vi "Begin.vi"() -> (0 "error out":errorcluster)   [LabVIEW 2013]
doc: "Called before other user functions, this VI is expected to open initial I/O refnums, load in file data, and do all program initialization. Notice that the <B>error out</B> terminal is simply used for data flow. Wiring it to other structures or subVIs ensures that this VI runs first."
uses:
  <vilib>/Rock Robotics/WPI/DriverStation/WPI_DriverStationRobotMode2.ctl
  <vilib>/Rock Robotics/WPI/Relay/WPI_RelayDirection.ctl
  <vilib>/Rock Robotics/SystemInterfaces/Typedef/FPGA_TypedefDigitalModule.ctl
  <vilib>/Rock Robotics/WPI/SafetyOutput/WPI_SafetyOutputConfigMenu.ctl
  <vilib>/Rock Robotics/WPI/Joystick/WPI_JoystickDeviceEnum.ctl
  <vilib>/Rock Robotics/SystemInterfaces/DIO/FPGA_DIOChannel.ctl
  <vilib>/Rock Robotics/WPI/Encoder/WPI_EncoderType.ctl
  <vilib>/Rock Robotics/SystemInterfaces/AI/FPGA_AIGyroChannel.ctl
  <vilib>/Rock Robotics/SystemInterfaces/Typedef/FPGA_TypedefAnalogModuleForGyro.ctl
  <vilib>/Rock Robotics/SystemInterfaces/DIO/FPGA_DIORelayChannel.ctl
  <vilib>/Rock Robotics/WPI/CAN/Jaguar/SubVIs/WPI_CANJaguar_ControlMode.ctl
  Robot Global Data.vi
  <vilib>/Rock Robotics/WPI/RobotDrive/WPI_RobotDriveOpen4MotorWithCANJaguar.vi
  <vilib>/Rock Robotics/WPI/Counter/WPI_CounterDigitalInputToDigitalSource.vi
  <vilib>/Rock Robotics/WPI/Counter/WPI_CounterOpen Semi Period Mode.vi
  <vilib>/Rock Robotics/WPI/MotorControl/WPI_MotorControlOpenCANJaguar.vi
panel:
  # "Launch Angle Position PID"
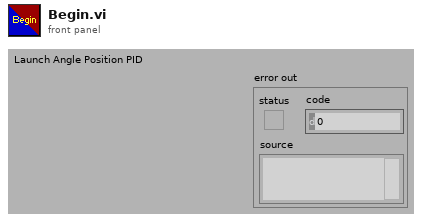
[diagram p1: front panel]
types:
  T1 = typedef "WPI_SafetyOutputConfigMenu.ctl" = enum16{"Enable", "Disable"}
  T2 = typedef "FPGA_TypedefDigitalModule.ctl" = enum16{"Digital Module 1", "Digital Module 2"}
  T3 = typedef "WPI_RelayDirection.ctl" = enum16{"Both directions", "Forward only", "Reverse only"}
  T4 = typedef "WPI_DriverStationRobotMode2.ctl" = enum16{"Autonomous Disabled", "Autonomous Enabled", "Teleop Disabled", "Teleop Enabled", "Timeout", "Finish", "Test Disabled", "Test Enabled"}
  T5 = typedef "WPI_JoystickDeviceEnum.ctl" = enum16{"USB 1", "USB 2", "USB 3", "USB 4", "Kinect 1", "Kinect 2"}
  T6 = typedef "FPGA_DIOChannel.ctl" = enum8{"DIO 1", "DIO 2", "DIO 3", "DIO 4", "DIO 5", "DIO 6", "DIO 7", "DIO 8", "DIO 9", "DIO 10", "DIO 11", "DIO 12", "DIO 13", "DIO 14", "Invalid"}
  T7 = typedef "FPGA_TypedefAnalogModuleForGyro.ctl" = enum16{"Analog Module 1"}
  T8 = typedef "FPGA_AIGyroChannel.ctl" = enum8{"AI 1", "AI 2", "Invalid"}
  T9 = typedef "FPGA_DIORelayChannel.ctl" = enum8{"Relay 1", "Relay 2", "Relay 3", "Relay 4", "Relay 5", "Relay 6", "Relay 7", "Relay 8", "Invalid"}
  T10 = typedef "WPI_CANJaguar_ControlMode.ctl" = enum8{"Percent VBus", "Current", "Speed", "Position", "Voltage"}
  T11 = typedef "WPI_JoystickDevRef.ctl" = cluster{"Device":T5}
  T12 = typedef "WPI_RobotDriveDevRef.ctl" = cluster{"DevStatus":errorcluster, "Motors[]":T13[], "Square Inputs":bool, "Max Output":dbl, "Isochronous":bool}
  T13 = typedef "WPI_MotorControlDeviceRef.ctl" = cluster{"DeviceStatus":errorcluster, "Type":enum16{"PWM", "CAN"}, "PWM":cluster{"Digital Module":T2, "PWM Channel":T14, "DeadBand":T15}, "CAN":cluster{"Device Number":u8, "Control Mode":T10, "Semaphore":T16, "Max Vout":dbl}, "Invert":bool, "TransformRef":T17, "InvTransformRef":T17}
  T14 = typedef "FPGA_DIOPWMChannel.ctl" = enum8{"PWM 1", "PWM 2", "PWM 3", "PWM 4", "PWM 5", "PWM 6", "PWM 7", "PWM 8", "PWM 9", "PWM 10", "Invalid"}
  T15 = typedef "WPI_PWMDeadband.ctl" = cluster{"Name":string, "maxPositivePwm":i32, "minPositivePwm":i32, "centerPwm":i32, "maxNegativePwm":i32, "minNegativePwm":i32, "angularRange":u16}
  T16 = typedef "Semaphore RefNum" = refnum<k1>
  T17 = typedef "WPI_PWMTransform_ConPane.ctl" = refnum<vi>
  T18 = typedef "WPI_EncoderType.ctl" = enum16{"1x", "2x", "4x"}
  T19 = typedef "WPI_DigitalInputDevRef.ctl" = cluster{"DevStatus":errorcluster, "DIO Channel":T6, "Digital Module":T2}
  T20 = typedef "FPGA_CounterEncoderSourceConvertionLVSourceType.ctl" = cluster{"DevStatus":errorcluster, "AnalogTriggerMode?":bool, "DigitalMode":cluster{"Digital Module":T2, "DIO Channel":T21}, "AnalogTriggerMode":cluster{"AnalogTriggerIndex":T22, "OutputType":T23}}
  T21 = typedef "FPGA_DIODigitalSourceChannel.ctl" = enum8{"DIO 1", "DIO 2", "DIO 3", "DIO 4", "DIO 5", "DIO 6", "DIO 7", "DIO 8", "DIO 9", "DIO 10", "DIO 11", "DIO 12", "DIO 13", "DIO 14", "Disabled"}
  T22 = typedef "FPGA_AnalogTriggerIndex.ctl" = enum8{"Trig 0", "Trig 1", "Trig 2", "Trig 3", "Trig 4", "Trig 5", "Trig 6", "Trig 7", "Invalid"}
  T23 = typedef "FPGA_AnalogTriggerOutType.ctl" = enum16{"InWindow", "TriggerState", "Rising", "Falling"}
  T24 = typedef "WPI_EncoderDevRef.ctl" = cluster{"DevStatus":errorcluster, "EncoderIndex":T25, "CounterIndex":T26, "DistancePerCount":dbl, "Decoding Type":T18}
  T25 = typedef "FPGA_EncoderIdx.ctl" = enum8{"Enc 0", "Enc 1", "Enc 2", "Enc 3", "Invalid"}
  T26 = typedef "FPGA_CounterCtrSystemIndex.ctl" = enum8{"Ctr 0", "Ctr 1", "Ctr 2", "Ctr 3", "Ctr 4", "Ctr 5", "Ctr 6", "Ctr 7", "Invalid"}
  T27 = typedef "WPI_GyroDevRef.ctl" = cluster{"DevStatus":errorcluster, "Analog Module":T28, "Analog Channel":T29, "Offset":dbl, "Gain (VoltsPerDegree/Second)":dbl}
  T28 = typedef "FPGA_TypedefAnalogModule.ctl" = enum16{"Analog Module 1", "Analog Module 2"}
  T29 = typedef "FPGA_AIChannel.ctl" = enum8{"AI 1", "AI 2", "AI 3", "AI 4", "AI 5", "AI 6", "AI 7", "AI 8", "Invalid"}
  T30 = typedef "WPI_CounterDevRef.ctl" = cluster{"DevStatus":errorcluster, "CntIndex":T26}
  T31 = typedef "WPI_RelayDevRef.ctl" = cluster{"DevStatus":errorcluster, "Relay Channel":T9, "Digital Module":T2, "Relay Direction":T3}
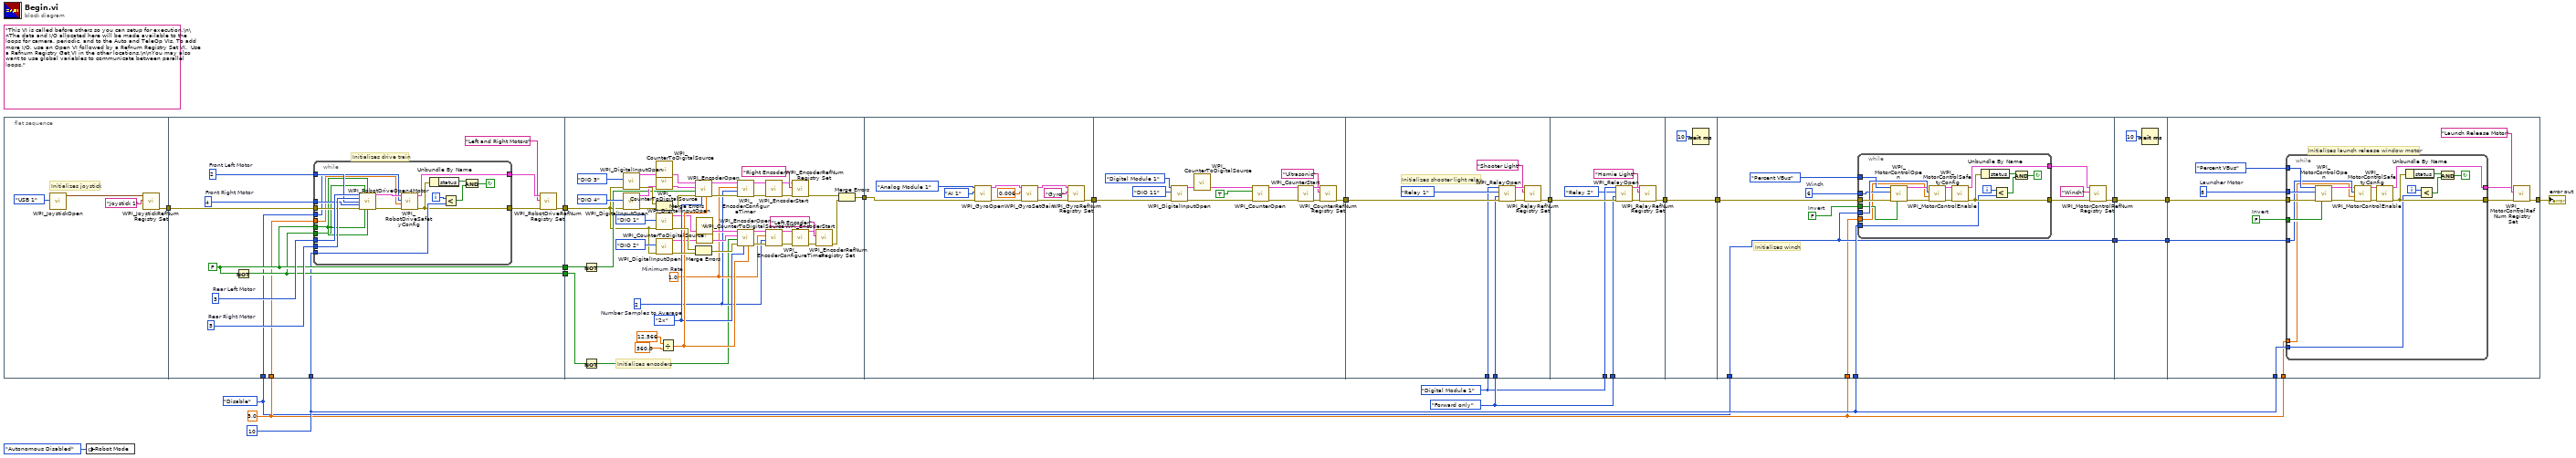
[diagram p0: block diagram]
diagram:
  w7 = WPI_SafetyOutputConfigMenu."Disable" ("mode")
  w8 = 3.0 ("timeout (s)")
  w3 = FPGA_TypedefDigitalModule."Digital Module 1" ("Digital Module (Module 1)")
  w4 = WPI_RelayDirection."Forward only" ("Relay Direction")
  w10 = 10 ("y")
  (unwired) "This VI is called before others so you can setup for execution.\n\nThe data and I/O allocated here will be made available to the loops for camera, periodic, and to the Auto and TeleOp VIs. To add more I/O, use an Open VI followed by a Refnum Registry Set VI.  Use a Refnum Registry Get VI in the other locations.\n\nYou may also want to use global variables to communicate between parallel loops."
  n1 = flat-sequence {
    tunnel: [w22] -> w21
    tunnel: w21 -> [w32]
    tunnel: [w31] -> w20
    tunnel: [w30] -> w19
    tunnel: [w29] -> w18
    tunnel: w10 -> [w28]
    tunnel: w8 -> [w27]
    tunnel: w7 -> [w26]
    tunnel: w18 -> [w63]
    tunnel: w19 -> [w62]
    tunnel: w20 -> [w61]
    tunnel: [w58] -> w9
    tunnel: [w107] -> w2
    tunnel: w9 -> [w113]
    tunnel: w2 -> [w120]
    tunnel: [w115] -> w1
    tunnel: w1 -> [w134]
    tunnel: w4 -> [w129]
    tunnel: w3 -> [w128]
    tunnel: [w127] -> w6
    tunnel: w6 -> [w139]
    tunnel: [w138] -> w5
    tunnel: w4 -> [w137]
    tunnel: w3 -> [w136]
    tunnel: [w143] -> w11
    tunnel: w5 -> [w143]
    tunnel: [w154] -> w15
    tunnel: [w146] -> w13
    tunnel: w10 -> [w151]
    tunnel: w11 -> [w147]
    tunnel: w7 -> [w146]
    tunnel: w8 -> [w145]
    tunnel: w15 -> [w175]
    tunnel: [w175] -> w14
    tunnel: w13 -> [w174]
    tunnel: [w174] -> w12
    tunnel: w14 -> [w182]
    tunnel: w12 -> [w181]
    tunnel: [w178] -> w16
    tunnel: w10 -> [w177]
    tunnel: w8 -> [w176]
    frame #0 {
      # "Initializes joystick"
      n2 = call <vilib>:"WPI_JoystickOpen.vi"("JoystickDevice"=WPI_JoystickDeviceEnum."USB 1") -> ("JoystickDevRef"=w24:T11)  [unwired: 10 in]
      n3 = call <vilib>:"WPI_JoystickRefNum Registry Set.vi"("refnum name"="Joystick 1", "JoystickDevRef"=w24) -> ("error out"=w22:errorcluster)  [unwired: 8 in, 1 out]
    }
    frame #1 {
      w30 = FALSE ("Rear Left Motor Inverted")
      w33 = u8 4  # Front Right Motor
      w34 = u8 2  # Front Left Motor
      w35 = u8 5  # Rear Right Motor
      w36 = u8 3  # Rear Left Motor
      # "Initializes drive train"
      n4 = Not(x=w30) -> (.not. x?=w29:bool)
      n5 = while {
        tunnel: [w44] -> w39
        tunnel: [w45] -> w38
        tunnel: w36 -> [w57]
        tunnel: w35 -> [w56]
        tunnel: w34 -> [w55]
        tunnel: w33 -> [w54]
        tunnel: w32 -> [w53]
        tunnel: w30 -> [w52]
        tunnel: w29 -> [w51]
        tunnel: w28 -> [w47]
        tunnel: w26 -> [w41]
        tunnel: w27 -> [w40]
        i -> [w48]
        stop <- w50 continue-if-true
        n6 = call-poly <vilib>:"WPI_RobotDriveOpen4Motor.vi"("Rear Left Motor"=w57, "Rear Left Motor Inverted"=w51, "Rear Right Motor Inverted"=w52, "Rear Right Motor"=w56, "Front Left Motor"=w55, "Front Right Motor"=w54, "error in (no error)"=w53, "Front Left Motor Inverted"=w51, "Front Right Motor Inverted"=w52) -> ("RobotDriveDevRef"=w43:T12, "error out"=w42:errorcluster)  [unwired: 5 in]
        n7 = call <vilib>:"WPI_RobotDriveSafetyConfig.vi"("error in (no error)"=w42, "timeout (s)"=w40, "mode"=w41, "RobotDriveDevRef"=w43) -> ("error out"=w44:errorcluster, "RobotDriveDevRef"=w45:T12)  [unwired: 6 in]
        n8 = Unbundle By Name(w44) -> ("status"=w49:bool)
        n9 = Less?(x=w48, y=w47) -> (x < y?=w46:bool)
        n10 = And(x=w49, y=w46) -> (x .and. y?=w50:bool)
      }
      n11 = call <vilib>:"WPI_RobotDriveRefNum Registry Set.vi"("error in (no error)"=w39, "refnum name"="Left and Right Motors", "RobotDriveDevRef"=w38) -> ("error out"=w31:errorcluster)  [unwired: 7 in, 1 out]
    }
    frame #2 {
      w71 = u8 2  # Number Samples to Average
      w72 = 1.0  # Minimum Rate
      w81 = WPI_EncoderType."2x" ("Decoding Type")
      # "Initializes encoders"
      n12 = Not(x=w62) -> (.not. x?=w65:bool)
      n13 = Not(x=w63) -> (.not. x?=w66:bool)
      n14 = call <vilib>:"WPI_DigitalInputOpen.vi"("error in (no error)"=w61, "DIO Channel"=FPGA_DIOChannel."DIO 3") -> ("error out"=w102:errorcluster, "DigitalInputDevRef"=w70:T19)  [unwired: 8 in]
      n15 = call <vilib>:"WPI_DigitalInputOpen.vi"("error in (no error)"=w61, "DIO Channel"=FPGA_DIOChannel."DIO 4") -> ("error out"=w101:errorcluster, "DigitalInputDevRef"=w69:T19)  [unwired: 8 in]
      n16 = Merge Errors(w102, w101) -> (w100:errorcluster)
      n17 = call-poly <vilib>:"WPI_CounterToDigitalSource.vi"("DigitalInputDevRef"=w70) -> ("Digital Source"=w103:T20)  [unwired: 6 in]
      n18 = call-poly <vilib>:"WPI_CounterToDigitalSource.vi"("DigitalInputDevRef"=w69) -> ("Digital Source"=w99:T20)  [unwired: 6 in]
      n19 = call <vilib>:"WPI_DigitalInputOpen.vi"("error in (no error)"=w61, "DIO Channel"=FPGA_DIOChannel."DIO 1") -> ("error out"=w97:errorcluster, "DigitalInputDevRef"=w67:T19)  [unwired: 8 in]
      n20 = call <vilib>:"WPI_DigitalInputOpen.vi"("error in (no error)"=w61, "DIO Channel"=FPGA_DIOChannel."DIO 2") -> ("error out"=w96:errorcluster, "DigitalInputDevRef"=w68:T19)  [unwired: 8 in]
      n21 = Divide(x=12.566, y=360.0) -> (x/y=w86:dbl)
      n22 = call <vilib>:"WPI_EncoderOpen.vi"("DistancePerCount"=w86, "Decoding Type"=w81, "error in (no error)"=w100, "Invert Direction (False)"=w65, "BSource"=w99, "ASource"=w103) -> ("error out"=w73:errorcluster, "EncoderDevRef"=w76:T24)  [unwired: 4 in]
      n23 = Merge Errors(w97, w96) -> (w95:errorcluster)
      n24 = call-poly <vilib>:"WPI_CounterToDigitalSource.vi"("DigitalInputDevRef"=w67) -> ("Digital Source"=w98:T20)  [unwired: 6 in]
      n25 = call-poly <vilib>:"WPI_CounterToDigitalSource.vi"("DigitalInputDevRef"=w68) -> ("Digital Source"=w94:T20)  [unwired: 6 in]
      n26 = call <vilib>:"WPI_EncoderConfigureTimer.vi"("error in (no error)"=w73, "Number Samples to Average"=w71, "Minimum Rate"=w72, "EncoderDevRef"=w76) -> ("error out"=w74:errorcluster, "EncoderDevRef"=w75:T24)  [unwired: 6 in]
      n27 = call <vilib>:"WPI_EncoderOpen.vi"("DistancePerCount"=w86, "Decoding Type"=w81, "error in (no error)"=w95, "Invert Direction (False)"=w66, "BSource"=w94, "ASource"=w98) -> ("error out"=w79:errorcluster, "EncoderDevRef"=w80:T24)  [unwired: 4 in]
      n28 = call <vilib>:"WPI_EncoderStart.vi"("error in (no error)"=w74, "EncoderDevRef"=w75) -> ("error out"=w82:errorcluster, "EncoderDevRef"=w83:T24)  [unwired: 8 in]
      n29 = call <vilib>:"WPI_EncoderConfigureTimer.vi"("error in (no error)"=w79, "Number Samples to Average"=w71, "Minimum Rate"=w72, "EncoderDevRef"=w80) -> ("error out"=w77:errorcluster, "EncoderDevRef"=w78:T24)  [unwired: 6 in]
      n30 = call <vilib>:"WPI_EncoderRefNum Registry Set.vi"("error in (no error)"=w82, "refnum name"="Right Encoder", "EncoderDevRef"=w83) -> ("error out"=w60:errorcluster)  [unwired: 7 in, 1 out]
      n31 = call <vilib>:"WPI_EncoderStart.vi"("error in (no error)"=w77, "EncoderDevRef"=w78) -> ("error out"=w84:errorcluster, "EncoderDevRef"=w85:T24)  [unwired: 8 in]
      n32 = call <vilib>:"WPI_EncoderRefNum Registry Set.vi"("error in (no error)"=w84, "refnum name"="Left Encoder", "EncoderDevRef"=w85) -> ("error out"=w59:errorcluster)  [unwired: 7 in, 1 out]
      n33 = Merge Errors(w60, w59) -> (w58:errorcluster)
    }
    frame #3 {
      n34 = call <vilib>:"WPI_GyroOpen.vi"("error in (no error)"=w113, "Analog Channel"=FPGA_AIGyroChannel."AI 1", "Analog Module (Module 1)"=FPGA_TypedefAnalogModuleForGyro."Analog Module 1") -> ("error out"=w110:errorcluster, "GyroDevRef"=w109:T27)  [unwired: 6 in, 1 out]
      n35 = call <vilib>:"WPI_GyroSetGain.vi"("error in (no error)"=w110, "Gain (VoltsPerDegree/Second)"=0.006, "GyroDevRef"=w109) -> ("error out"=w105:errorcluster, "GyroDevRef"=w106:T27)  [unwired: 7 in]
      n36 = call <vilib>:"WPI_GyroRefNum Registry Set.vi"("error in (no error)"=w105, "refnum name"="Gyro", "GyroDevRef"=w106) -> ("error out"=w107:errorcluster)  [unwired: 7 in, 1 out]
    }
    frame #4 {
      n37 = call <vilib>:"WPI_DigitalInputOpen.vi"("error in (no error)"=w120, "DIO Channel"=FPGA_DIOChannel."DIO 11", "Digital Module (Module 1)"=FPGA_TypedefDigitalModule."Digital Module 1") -> ("error out"=w121:errorcluster, "DigitalInputDevRef"=w125:T19)  [unwired: 7 out]
      n38 = call-poly <vilib>:"WPI_CounterToDigitalSource.vi"("DigitalInputDevRef"=w125) -> ("Digital Source"=w123:T20)  [unwired: 6 in]
      n39 = call-poly <vilib>:"WPI_CounterOpen.vi"("error in (no error)"=w121, "High Pulse (T)"=TRUE, "Source"=w123) -> ("error out"=w122:errorcluster, "CounterDevRef"=w124:T30)  [unwired: 7 in]
      n40 = call <vilib>:"WPI_CounterStart.vi"("error in (no error)"=w122, "CounterDevRef in"=w124) -> ("error out"=w117:errorcluster, "CounterDevRef out"=w116:T30)  [unwired: 8 in]
      n41 = call <vilib>:"WPI_CounterRefNum Registry Set.vi"("error in (no error)"=w117, "refnum name"="Ultrasonic", "CounterDevRef"=w116) -> ("error out"=w115:errorcluster)  [unwired: 7 in, 1 out]
    }
    frame #5 {
      # "Initializes shooter light relay"
      n42 = call <vilib>:"WPI_RelayOpen.vi"("error in (no error)"=w134, "Relay Direction"=w129, "Relay Channel"=FPGA_DIORelayChannel."Relay 1", "Digital Module (Module 1)"=w128) -> ("error out"=w133:errorcluster, "RelayDevRef"=w132:T31)  [unwired: 6 in]
      n43 = call <vilib>:"WPI_RelayRefNum Registry Set.vi"("error in (no error)"=w133, "refnum name"="Shooter Light", "RelayDevRef"=w132) -> ("error out"=w127:errorcluster)  [unwired: 7 in, 1 out]
    }
    frame #6 {
      n44 = call <vilib>:"WPI_RelayOpen.vi"("error in (no error)"=w139, "Relay Direction"=w137, "Relay Channel"=FPGA_DIORelayChannel."Relay 2", "Digital Module (Module 1)"=w136) -> ("error out"=w142:errorcluster, "RelayDevRef"=w141:T31)  [unwired: 6 in]
      n45 = call <vilib>:"WPI_RelayRefNum Registry Set.vi"("error in (no error)"=w142, "refnum name"="Homie Light", "RelayDevRef"=w141) -> ("error out"=w138:errorcluster)  [unwired: 7 in, 1 out]
    }
    frame #7 {
      n46 = Wait (ms)(milliseconds to wait=u32 10) -> ()  [unwired: 1 out]
    }
    frame #8 {
      w148 = FALSE  # Invert
      w149 = u8 6  # Winch
      # "Initializes winch"
      n47 = while {
        tunnel: w147 -> [w170]
        tunnel: w146 -> [w169]
        tunnel: [w165] -> w153
        tunnel: [w166] -> w152
        tunnel: w151 -> [w163]
        tunnel: WPI_CANJaguar_ControlMode."Percent VBus" ("Control Mode") -> [w159]
        tunnel: w149 -> [w158]
        tunnel: w148 -> [w157]
        tunnel: w145 -> [w156]
        i -> [w164]
        stop <- w160 continue-if-true
        n48 = call-poly <vilib>:"WPI_MotorControlOpen.vi"("Invert"=w157, "error in (no error)"=w170, "Device Number"=w158, "Control Mode"=w159) -> ("error out"=w167:errorcluster, "MotorControlDeviceRef"=w168:T13)  [unwired: 6 in]
        n49 = call <vilib>:"WPI_MotorControlSafetyConfig.vi"("error in (no error)"=w167, "timeout (s)"=w156, "mode"=w169, "MotorControlDevRef"=w168) -> ("error out"=w172:errorcluster, "MotorControlDevRef"=w171:T13)  [unwired: 6 in]
        n50 = call <vilib>:"WPI_MotorControlEnable.vi"("error in (no error)"=w172, "CAN Jaguar Ref"=w171) -> ("error out"=w165:errorcluster, "CAN Jaguar Ref Out"=w166:T13)  [unwired: 8 in]
        n51 = Unbundle By Name(w165) -> ("status"=w161:bool)
        n52 = Less?(x=w164, y=w163) -> (x < y?=w162:bool)
        n53 = And(x=w161, y=w162) -> (x .and. y?=w160:bool)
      }
      n54 = call <vilib>:"WPI_MotorControlRefNum Registry Set.vi"("error in (no error)"=w153, "refnum name"="Winch", "MotorControlDevRef"=w152) -> ("error out"=w154:errorcluster)  [unwired: 7 in, 1 out]
    }
    frame #9 {
      n55 = Wait (ms)(milliseconds to wait=u32 10) -> ()  [unwired: 1 out]
    }
    frame #10 {
      w185 = u8 8  # Launcher Motor
      w186 = FALSE  # Invert
      # "Initializes launch release window motor"
      n56 = while {
        tunnel: w186 -> [w203]
        tunnel: w185 -> [w202]
        tunnel: WPI_CANJaguar_ControlMode."Percent VBus" ("Control Mode") -> [w201]
        tunnel: w182 -> [w198]
        tunnel: w181 -> [w197]
        tunnel: [w190] -> w180
        tunnel: [w194] -> w179
        tunnel: w177 -> [w188]
        tunnel: w176 -> [w187]
        i -> [w189]
        stop <- w193 continue-if-true
        n57 = call-poly <vilib>:"WPI_MotorControlOpen.vi"("Invert"=w203, "error in (no error)"=w198, "Device Number"=w202, "Control Mode"=w201) -> ("error out"=w195:errorcluster, "MotorControlDeviceRef"=w196:T13)  [unwired: 6 in]
        n58 = call <vilib>:"WPI_MotorControlSafetyConfig.vi"("error in (no error)"=w195, "timeout (s)"=w187, "mode"=w197, "MotorControlDevRef"=w196) -> ("error out"=w200:errorcluster, "MotorControlDevRef"=w199:T13)  [unwired: 6 in]
        n59 = call <vilib>:"WPI_MotorControlEnable.vi"("error in (no error)"=w200, "CAN Jaguar Ref"=w199) -> ("error out"=w190:errorcluster, "CAN Jaguar Ref Out"=w194:T13)  [unwired: 8 in]
        n60 = Unbundle By Name(w190) -> ("status"=w191:bool)
        n61 = Less?(x=w189, y=w188) -> (x < y?=w192:bool)
        n62 = And(x=w191, y=w192) -> (x .and. y?=w193:bool)
      }
      n63 = call <vilib>:"WPI_MotorControlRefNum Registry Set.vi"("error in (no error)"=w180, "refnum name"="Launch Release Motor", "MotorControlDevRef"=w179) -> ("error out"=w178:errorcluster)  [unwired: 7 in, 1 out]
    }
  }
  n64 = global write "Robot Global Data.vi" "Robot Mode"(WPI_DriverStationRobotMode2."Autonomous Disabled" ("Robot Mode")) -> ()
  "error out" <- w16
